vi "TCP Check Connection.vi"(8 "error in (no error)":errorcluster, 11 "Connection In":T1) -> (0 "error out":errorcluster, 2 "Disconnected":bool, 3 "Connection out":T1)   [LabVIEW 2010]
doc: "This VI removes the host connection from the connection manager list if it becomes disconnected for any reason.\n\nCopyright 2015, 2016, 2017 National Instruments Corporation\n\nLicensed under the Apache License, Version 2.0 (the \"License\"); you may not use this file except in compliance with the License.\n\n You may obtain a copy of the License at\n\n http://www.apache.org/licenses/LICENSE-2.0\n\nUnless required by applicable law or agreed to in writing, software distributed under the License is distributed on an \"AS IS\" BASIS, WITHOUT WARRANTIES OR CONDITIONS OF ANY KIND, either express or implied.\n\nSee the License for the specific language governing permissions and limitations under the License."
uses:
  stm_TCP Connection Info.ctl
  stm_MetaDataElement.ctl
  Connection Manager/TCP/TCP Connection Manager.vi
  NI STM.lvlib
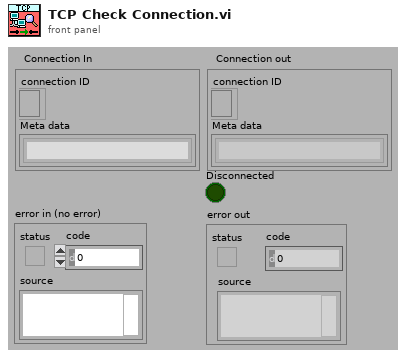
[diagram p1: front panel]
types:
  T1 = typedef "stm_TCP Connection Info.ctl" = cluster{"connection ID":refnum<k5>, "Meta data":T2[]}
  T2 = typedef "stm_MetaDataElement.ctl" = string
  T3 = typedef "NI STM.lvlib/TCP Connection Info.ctl" = cluster{"connection ID":refnum<k5>, "meta data":T4[]}
  T4 = typedef "NI STM.lvlib/MetaDataElement.ctl" = string
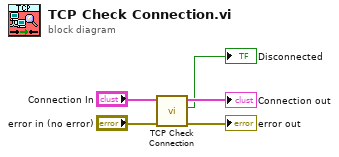
[diagram p0: block diagram]
diagram:
  n1 = call "TCP Check Connection.vi"("error in"="error in (no error)", "connection in"="Connection In") -> ("error out"=→"error out":errorcluster, "disconnected?"=→"Disconnected":bool, "connection out"=→"Connection out":T3)  [unwired: 7 in]
